vi "ex_RemoveLastChar.vi"(2 "Search":string="0", 3 "String":string) -> (0 "Found":bool, 1 "Result":string)   [LabVIEW 2017]
doc: "Removes the last character from a string if it matches the search character."
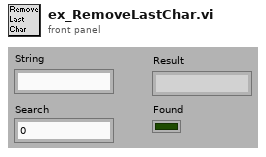
[diagram p1: front panel]
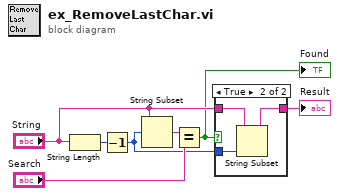
[diagram p0: block diagram]
diagram:
  n1 = String Length(string="String") -> (length=w7:i32)
  n2 = Decrement(x=w7) -> (x-1=w3:i32)
  n3 = String Subset(string="String", offset (0)=w3) -> (substring=w5:string)  [unwired: 1 in]
  n4 = Equal?(x=w5, y="Search") -> (x = y?=w1:bool)
  "Found" <- w1
  n5 = case shown="True" w1 {
    tunnel: "String" -> [w8 w11]
    tunnel: [w8 w9] -> w2
    tunnel: w3 -> [_ w10]
    frame False {
    }
    frame True {
      n6 = String Subset(string=w11, length (rest)=w10) -> (substring=w9:string)  [unwired: 1 in]
    }
  }
  "Result" <- w2
